vi "Simula stato PLC_3.vi"(11 "USCITE PLC":T1) -> (3 "STATO PLC":T4)   [LabVIEW 2019]
uses:
  STATO PLC 3.ctl
  Uscite PLC 3.ctl
  controls/statoAO_plc_3.ctl
  StatoDO_PLC_3.ctl
panel:
  in  "Stato DI_PLC.Reset da pulsantiera":bool
  in  "Stato DI_PLC.Stop da pulsantiera":bool
  in  "Stato DI_PLC.Start da pulsantiera":bool
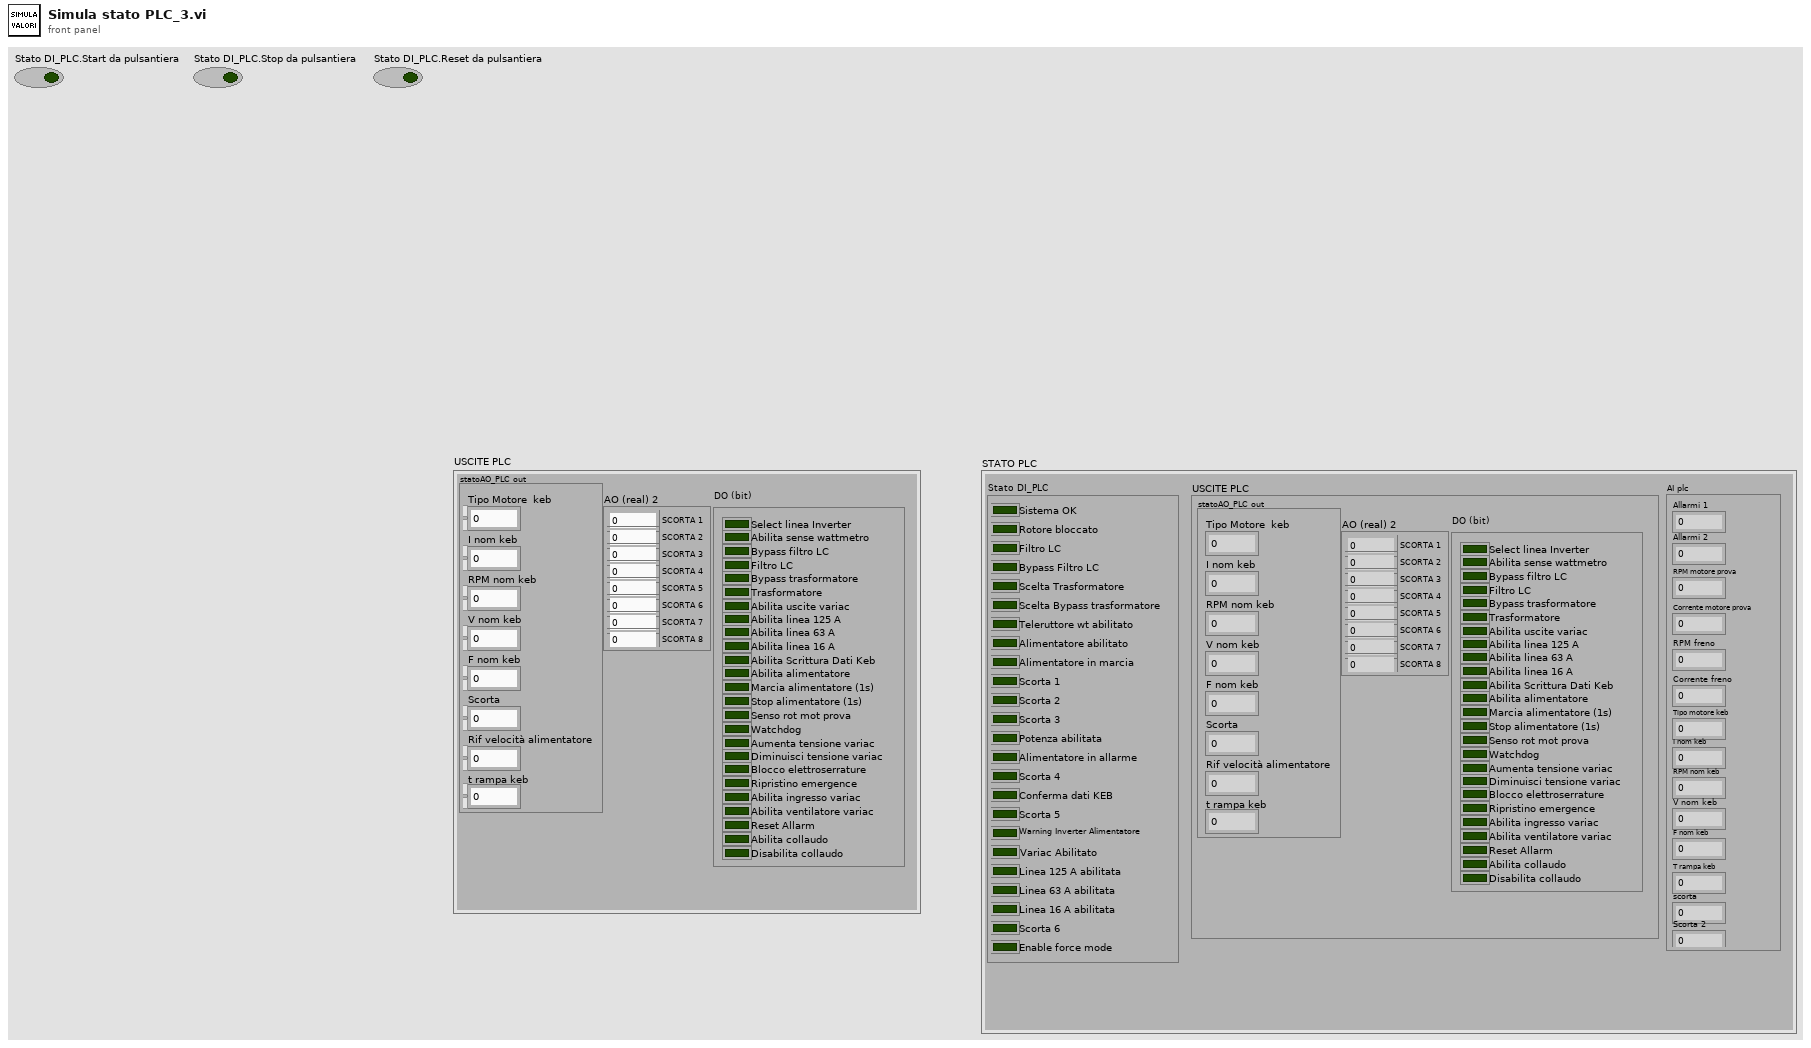
[diagram p1: front panel]
types:
  T1 = typedef "Uscite PLC 3.ctl" = cluster{"AO (real) 2":cluster{"SCORTA 1":dbl, "SCORTA 2":dbl, "SCORTA 3":dbl, "SCORTA 4":dbl, "SCORTA 5":dbl, "SCORTA 6":dbl, "SCORTA 7":dbl, "SCORTA 8":dbl}, "statoAO_PLC out":T2, "DO (bit)":T3}
  T2 = typedef "statoAO_plc_3.ctl" = cluster{"Rif velocità alimentatore":dbl, "Scorta":dbl, "Tipo Motore  keb":dbl, "I nom keb":dbl, "RPM nom keb":dbl, "V nom keb":dbl, "F nom keb":dbl, "t rampa keb":dbl}
  T3 = typedef "StatoDO_PLC_3.ctl" = cluster{"Select linea Inverter":bool, "Abilita sense wattmetro":bool, "Bypass filtro LC":bool, "Filtro LC":bool, "Bypass trasformatore":bool, "Trasformatore":bool, "Abilita uscite variac":bool, "Abilita linea 125 A":bool, "Abilita linea 63 A":bool, "Abilita linea 16 A":bool, "Abilita Scrittura Dati Keb":bool, "Abilita alimentatore":bool, "Marcia alimentatore (1s)":bool, "Stop alimentatore (1s)":bool, "Senso rot mot prova":bool, "Watchdog":bool, "Aumenta tensione variac":bool, "Diminuisci tensione variac ":bool, "Blocco elettroserrature":bool, "Ripristino emergence":bool, "Abilita ingresso variac":bool, "Abilita ventilatore variac":bool, "Reset Allarm":bool, "Scorta 1":bool, "Scorta 2":bool, "Scorta 3":bool, "Scorta 4":bool, "Scorta 5":bool, "Scorta 6":bool, "Scorta 7":bool, "Scorta 8":bool, "Scorta 9":bool, "Abilita collaudo":bool, "Disabilita collaudo ":bool, "Scorta 10":bool, "Scorta 11":bool, "Scorta 12":bool, "Scorta 13":bool, "Scorta 14":bool, "Scorta 15":bool}
  T4 = typedef "STATO PLC 3.ctl" = cluster{"USCITE PLC":T1, "Stato DI_PLC":cluster{"Sistema OK":bool, "Rotore bloccato":bool, "Filtro LC":bool, "Bypass Filtro LC":bool, "Scelta Trasformatore":bool, "Scelta Bypass trasformatore":bool, "Teleruttore wt abilitato":bool, "Alimentatore abilitato":bool, "Alimentatore in marcia":bool, "Scorta 1":bool, "Scorta 2":bool, "Scorta 3":bool, "Potenza abilitata":bool, "Alimentatore in allarme":bool, "Scorta 4":bool, "Conferma dati KEB":bool, "Scorta 5":bool, "Warning Inverter Alimentatore":bool, "Variac Abilitato":bool, "Linea 125 A abilitata":bool, "Linea 63 A abilitata":bool, "Linea 16 A abilitata":bool, "Scorta 6":bool, "Enable force mode":bool}, "AI plc":cluster{"Allarmi 1":dbl, "Allarmi 2":dbl, "RPM motore prova":dbl, "Corrente motore prova":dbl, "RPM freno":dbl, "Corrente freno":dbl, "Tipo motore keb":dbl, "I nom keb":dbl, "RPM nom keb":dbl, "V nom keb":dbl, "F nom keb":dbl, "T rampa keb":dbl, "scorta":dbl, "Scorta 2":dbl}}
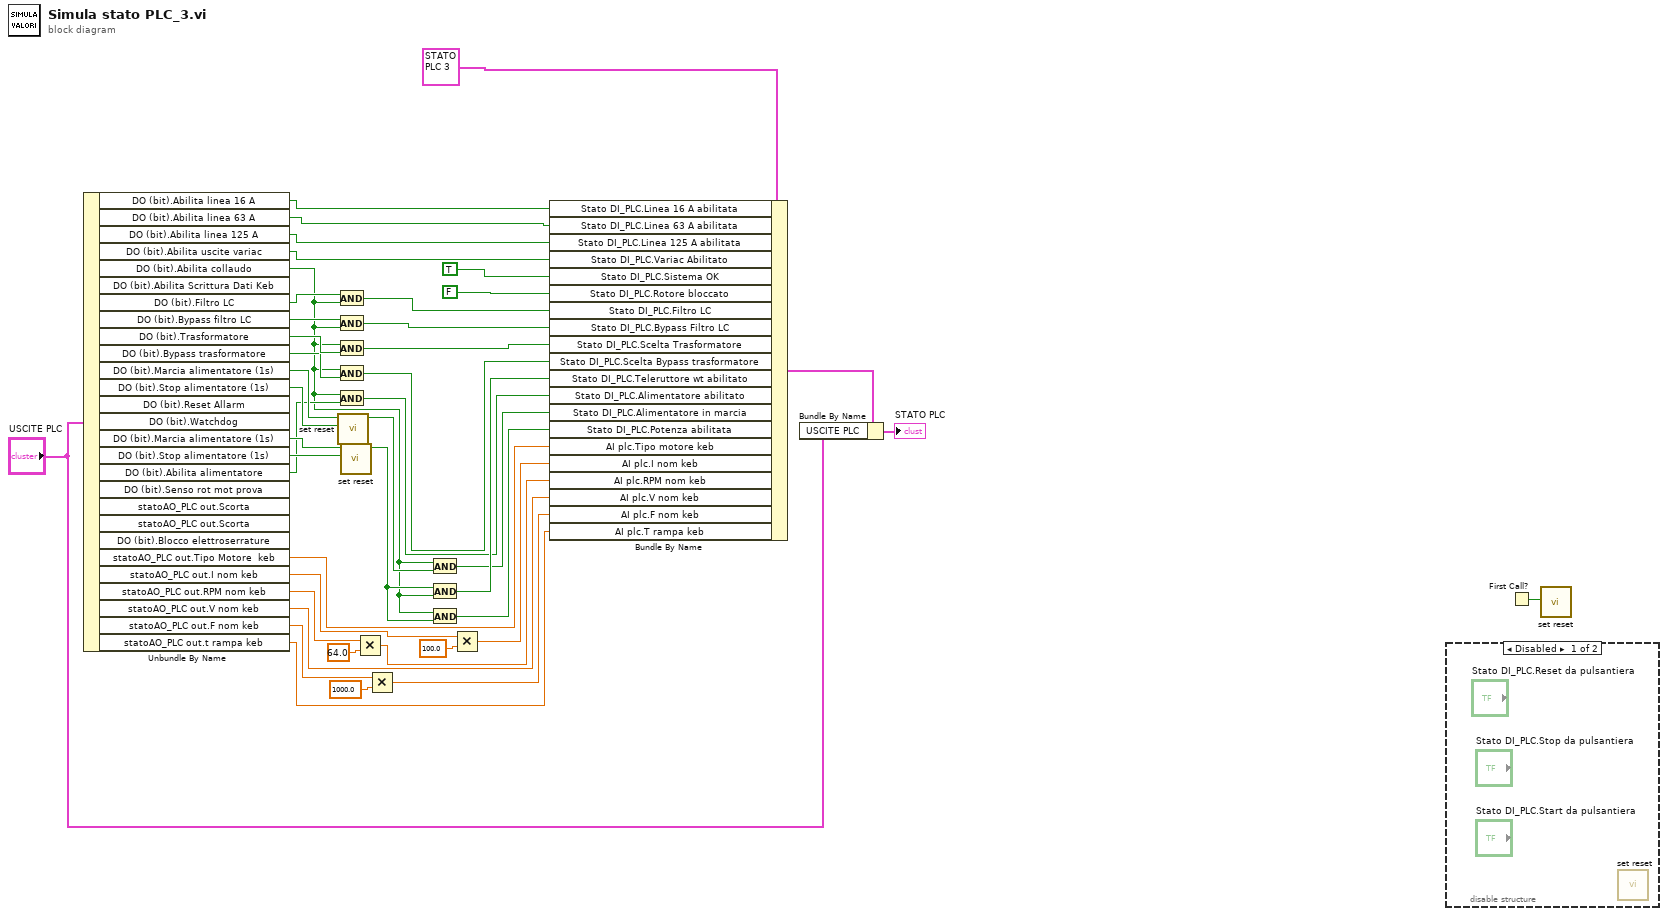
[diagram p0: block diagram]
diagram:
  n1 = Unbundle By Name("USCITE PLC") -> ("DO (bit).Abilita linea 16 A"=w4:bool, "DO (bit).Abilita linea 63 A"=w3:bool, "DO (bit).Abilita linea 125 A"=w2:bool, "DO (bit).Abilita uscite variac"=w5:bool, "DO (bit).Abilita collaudo"=w1:bool, "DO (bit).Filtro LC"=w36:bool, "DO (bit).Bypass filtro LC"=w35:bool, "DO (bit).Trasformatore"=w34:bool, "DO (bit).Bypass trasformatore"=w33:bool, "DO (bit).Marcia alimentatore (1s)"=w32:bool, "DO (bit).Stop alimentatore (1s)"=w31:bool, "DO (bit).Marcia alimentatore (1s)"=w29:bool, "DO (bit).Stop alimentatore (1s)"=w28:bool, "DO (bit).Abilita alimentatore"=w27:bool, "statoAO_PLC out.Tipo Motore  keb"=w26:dbl, "statoAO_PLC out.I nom keb"=w11:dbl, "statoAO_PLC out.RPM nom keb"=w9:dbl, "statoAO_PLC out.V nom keb"=w25:dbl, "statoAO_PLC out.F nom keb"=w7:dbl, "statoAO_PLC out.t rampa keb"=w24:dbl)  [unwired: 7 out]
  n2 = And(x=w36, y=w1) -> (x .and. y?=w23:bool)
  n3 = And(x=w35, y=w1) -> (x .and. y?=w22:bool)
  n4 = And(x=w1, y=w34) -> (x .and. y?=w21:bool)
  n5 = And(x=w1, y=w33) -> (x .and. y?=w20:bool)
  n6 = And(x=w1, y=w27) -> (x .and. y?=w18:bool)
  n7 = call "set reset.vi"("reset"=w31, "set"=w32) -> ("Boolean"=w30:bool)  [unwired: 9 in]
  n8 = call "set reset.vi"("reset"=w28, "set"=w29) -> ("Boolean"=w15:bool)  [unwired: 9 in]
  n9 = Multiply(x=w9, y=64.0) -> (x*y=w8:dbl)
  n10 = Multiply(x=w7, y=1000.0) -> (x*y=w6:dbl)
  n11 = And(x=w1, y=w30) -> (x .and. y?=w17:bool)
  n12 = And(x=w15, y=w1) -> (x .and. y?=w19:bool)
  n13 = And(x=w1, y=w15) -> (x .and. y?=w16:bool)
  n14 = Multiply(x=w11, y=100.0) -> (x*y=w10:dbl)
  n15 = Bundle By Name(cluster=T4 {"USCITE PLC"={"AO (real) 2"={"SCORTA 1"=0.0, "SCORTA 2"=0.0, "SCORTA 3"=0.0, "SCORTA 4"=0.0, "SCORTA 5"=0.0, "SCORTA 6"=0.0, "SCORTA 7"=0.0, "SCORTA 8"=0.0}, "statoAO_PLC out"={"Rif velocità alimentatore"=0.0, "Scorta"=0.0, "Tipo Motore  keb"=0.0, "I nom keb"=0.0, "RPM nom keb"=0.0, "V nom keb"=0.0, "F nom keb"=0.0, "t rampa keb"=0.0}, "DO (bit)"={"Select linea Inverter"=FALSE, "Abilita sense wattmetro"=FALSE, "Bypass filtro LC"=FALSE, "Filtro LC"=FALSE, "Bypass trasformatore"=FALSE, "Trasformatore"=FALSE, "Abilita uscite variac"=FALSE, "Abilita linea 125 A"=FALSE, "Abilita linea 63 A"=FALSE, "Abilita linea 16 A"=FALSE, "Abilita Scrittura Dati Keb"=FALSE, "Abilita alimentatore"=FALSE, "Marcia alimentatore (1s)"=FALSE, "Stop alimentatore (1s)"=FALSE, "Senso rot mot prova"=FALSE, "Watchdog"=FALSE, "Aumenta tensione variac"=FALSE, "Diminuisci tensione variac "=FALSE, "Blocco elettroserrature"=FALSE, "Ripristino emergence"=FALSE, "Abilita ingresso variac"=FALSE, "Abilita ventilatore variac"=FALSE, "Reset Allarm"=FALSE, "Scorta 1"=FALSE, "Scorta 2"=FALSE, "Scorta 3"=FALSE, "Scorta 4"=FALSE, "Scorta 5"=FALSE, "Scorta 6"=FALSE, "Scorta 7"=FALSE, "Scorta 8"=FALSE, "Scorta 9"=FALSE, "Abilita collaudo"=FALSE, "Disabilita collaudo "=FALSE, "Scorta 10"=FALSE, "Scorta 11"=FALSE, "Scorta 12"=FALSE, "Scorta 13"=FALSE, "Scorta 14"=FALSE, "Scorta 15"=FALSE}}, "Stato DI_PLC"={"Sistema OK"=FALSE, "Rotore bloccato"=FALSE, "Filtro LC"=FALSE, "Bypass Filtro LC"=FALSE, "Scelta Trasformatore"=FALSE, "Scelta Bypass trasformatore"=FALSE, "Teleruttore wt abilitato"=FALSE, "Alimentatore abilitato"=FALSE, "Alimentatore in marcia"=FALSE, "Scorta 1"=FALSE, "Scorta 2"=FALSE, "Scorta 3"=FALSE, "Potenza abilitata"=FALSE, "Alimentatore in allarme"=FALSE, "Scorta 4"=FALSE, "Conferma dati KEB"=FALSE, "Scorta 5"=FALSE, "Warning Inverter Alimentatore"=FALSE, "Variac Abilitato"=FALSE, "Linea 125 A abilitata"=FALSE, "Linea 63 A abilitata"=FALSE, "Linea 16 A abilitata"=FALSE, "Scorta 6"=FALSE, "Enable force mode"=FALSE}, "AI plc"={"Allarmi 1"=0.0, "Allarmi 2"=0.0, "RPM motore prova"=0.0, "Corrente motore prova"=0.0, "RPM freno"=0.0, "Corrente freno"=0.0, "Tipo motore keb"=0.0, "I nom keb"=0.0, "RPM nom keb"=0.0, "V nom keb"=0.0, "F nom keb"=0.0, "T rampa keb"=0.0, "scorta"=0.0, "Scorta 2"=0.0}} ("STATO PLC 2"), "Stato DI_PLC.Linea 16 A abilitata"=w4, "Stato DI_PLC.Linea 63 A abilitata"=w3, "Stato DI_PLC.Linea 125 A abilitata"=w2, "Stato DI_PLC.Variac Abilitato"=w5, "Stato DI_PLC.Sistema OK"=TRUE ("Stato DI_PLC.Locale\\Remoto"), "Stato DI_PLC.Rotore bloccato"=FALSE, "Stato DI_PLC.Filtro LC"=w23, "Stato DI_PLC.Bypass Filtro LC"=w22, "Stato DI_PLC.Scelta Trasformatore"=w21, "Stato DI_PLC.Scelta Bypass trasformatore"=w20, "Stato DI_PLC.Teleruttore wt abilitato"=w19, "Stato DI_PLC.Alimentatore abilitato"=w18, "Stato DI_PLC.Alimentatore in marcia"=w17, "Stato DI_PLC.Potenza abilitata"=w16, "AI plc.Tipo motore keb"=w26, "AI plc.I nom keb"=w10, "AI plc.RPM nom keb"=w8, "AI plc.V nom keb"=w25, "AI plc.F nom keb"=w6, "AI plc.T rampa keb"=w24) -> (w43:T4)
  n16 = Bundle By Name(cluster=w43, "USCITE PLC"="USCITE PLC") -> (→"STATO PLC":T4)
  n17 = disable-structure shown="Disabled" {
    frame Disabled {
      n18 = call "set reset.vi"() -> ()  [unwired: 11 in, 1 out]
    }
    frame Enabled {
    }
  }
  n19 = First Call?() -> (First Call?: T/F=w38:bool)
  n20 = call "set reset.vi"("reset"=w38) -> ()  [unwired: 10 in, 1 out]
